vi "GetParam.vi"(8 "error in (no error)":errorcluster caption="entrée d'erreur (pas d'erreur)", 11 "RobustScaler.lvclass":refnum<class "RobustScaler.lvclass">) -> (0 "error out":errorcluster caption="sortie d'erreur", 2 "RobustScaler":T1={"with_centering"=TRUE, "with_scaling"=TRUE, "quantile_range"={"q_min"=25.0, "q_max"=75.0}, "copy"=TRUE}, 3 "RobustScaler.lvclass":refnum<class "RobustScaler.lvclass">)   [LabVIEW 2020, in "RobustScaler.lvclass"]
doc: "Get Parameters"
uses:
  RobustScaler.lvclass
  RobustScaler.lvclass/RobustScaler.ctl
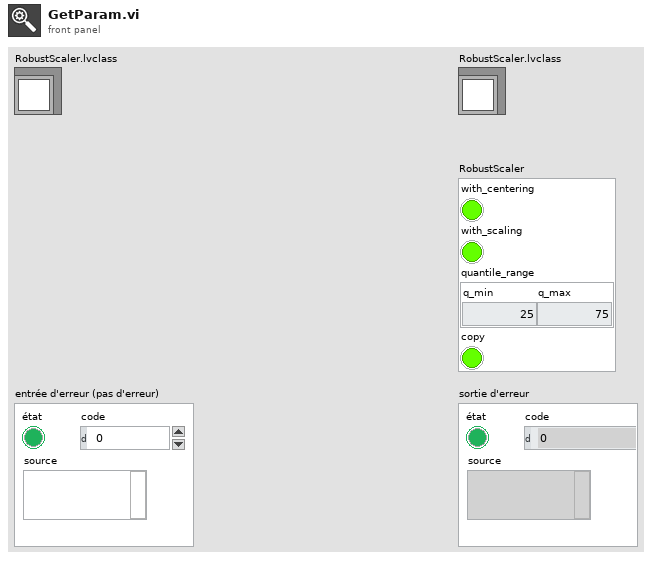
[diagram p1: front panel]
types:
  T1 = cluster{"with_centering":bool, "with_scaling":bool, "quantile_range":cluster{"q_min":dbl, "q_max":dbl}, "copy":bool}
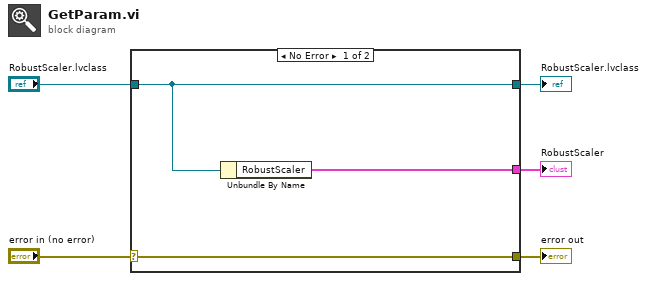
[diagram p0: block diagram]
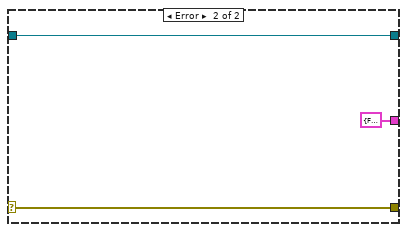
[diagram p2: hidden frame]
diagram:
  n1 = case shown="No Error" "error in (no error)" {
    selector: "error in (no error)" -> [w8 w10]
    tunnel: [w8 w10] -> w4
    tunnel: [w7 w11] -> w2
    tunnel: "RobustScaler.lvclass" -> [w7 w11]
    tunnel: [w6 T1 {"with_centering"=FALSE, "with_scaling"=FALSE, "quantile_range"={"q_min"=0.0, "q_max"=0.0}, "copy"=FALSE} ("RobustScaler")] -> w1
    frame No Error {
      n2 = Unbundle By Name(w7) -> ("RobustScaler"=w6:T1)
    }
    frame Error {
    }
  }
  "error out" <- w4
  "RobustScaler.lvclass" <- w2
  "RobustScaler" <- w1
